vi "GetColorFilePath.vi"(11 "String":string) -> (0 "name":string, 3 "path":path)   [LabVIEW 2022 SP3]
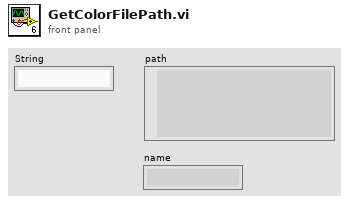
[diagram p1: front panel]
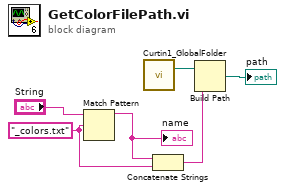
[diagram p0: block diagram]
diagram:
  w3 = "_colors.txt" ("pattern")
  n1 = Match Pattern(string="String", regular expression=w3) -> (before substring=w4:string)  [unwired: 1 in, 3 out]
  "name" <- w4
  n2 = call "Curtin1_GlobalFolder.vi"() -> ("LabVIEW Data Path"=w1:path)  [unwired: 1 in, 1 out]
  n3 = Concatenate Strings(w4, w3) -> (w6:string)
  n4 = Build Path(base path=w1, name or relative path=w6) -> (appended path=→"path":path)
